vi "ADC2ArrayEEG.vi"(0 "Numeric 6":i32, 2 "Numeric 5":i32, 4 "Numeric 4":i32, 5 "Numeric 3":i32, 8 "Numeric 7":i32, 9 "Numeric 2":i32, 12 "Numeric 8":i32, 13 "Numeric":i32, 17 "Numeric 9":i32) -> (10 "Numeric 8 out":dbl, 11 "Numeric 4 out":dbl, 14 "Numeric 7 out":dbl, 15 "Numeric 3 out":dbl, 16 "Numeric 6 out":dbl, 18 "Numeric 5 out":dbl, 19 "Numeric 2 out":dbl)   [LabVIEW 2021]
panel:
  out "Numeric 9 out":dbl
  out "Numeric out":dbl
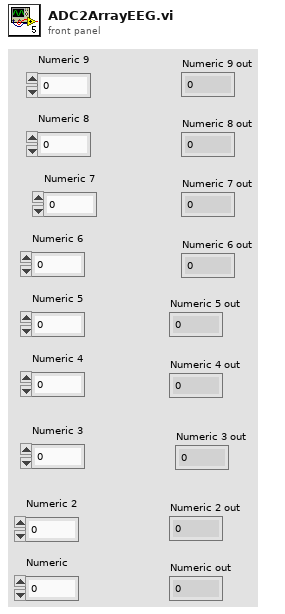
[diagram p1: front panel]
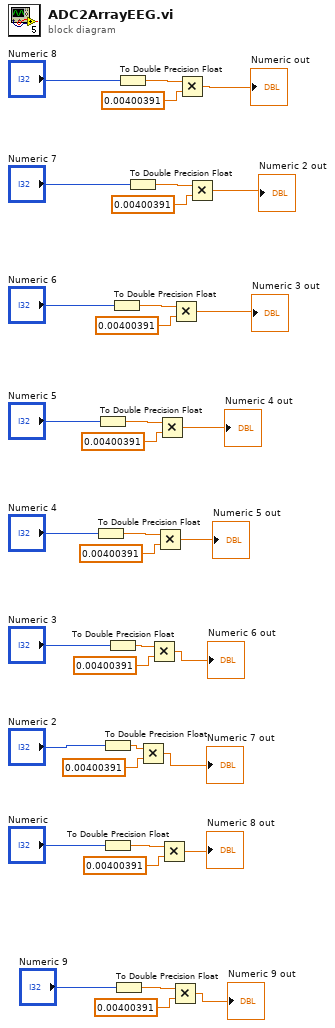
[diagram p0: block diagram]
diagram:
  n1 = To Double Precision Float(number="Numeric 4") -> (double precision float=w25:dbl)
  n2 = To Double Precision Float(number="Numeric 5") -> (double precision float=w22:dbl)
  n3 = To Double Precision Float(number="Numeric 2") -> (double precision float=w30:dbl)
  n4 = To Double Precision Float(number="Numeric") -> (double precision float=w32:dbl)
  n5 = To Double Precision Float(number="Numeric 3") -> (double precision float=w28:dbl)
  n6 = To Double Precision Float(number="Numeric 6") -> (double precision float=w19:dbl)
  n7 = To Double Precision Float(number="Numeric 9") -> (double precision float=w10:dbl)
  n8 = To Double Precision Float(number="Numeric 8") -> (double precision float=w13:dbl)
  n9 = To Double Precision Float(number="Numeric 7") -> (double precision float=w16:dbl)
  n10 = Multiply(x=w30, y=0.00400391) -> (x*y=→"Numeric 7 out":dbl)
  n11 = Multiply(x=w28, y=0.00400391) -> (x*y=→"Numeric 6 out":dbl)
  n12 = Multiply(x=w25, y=0.00400391) -> (x*y=→"Numeric 5 out":dbl)
  n13 = Multiply(x=w22, y=0.00400391) -> (x*y=→"Numeric 4 out":dbl)
  n14 = Multiply(x=w32, y=0.00400391) -> (x*y=→"Numeric 8 out":dbl)
  n15 = Multiply(x=w10, y=0.00400391) -> (x*y=→"Numeric 9 out":dbl)
  n16 = Multiply(x=w19, y=0.00400391) -> (x*y=→"Numeric 3 out":dbl)
  n17 = Multiply(x=w13, y=0.00400391) -> (x*y=→"Numeric out":dbl)
  n18 = Multiply(x=w16, y=0.00400391) -> (x*y=→"Numeric 2 out":dbl)
